vi "M3102A get data.vi"(5 "channel number":i32, 6 "TimeOut":i32, 7 "DAQpoints":i32, 8 "errorIn":errorcluster, 11 "moduleID":i32) -> (0 "errorOut":errorcluster, 2 "DAQdata":i16[](array[numeric]), 3 "moduleIDout":i32)   [LabVIEW 2021]
uses:
  <vilib>/Keysight_SD1/DAQ/base/DAQread_AIN.vi
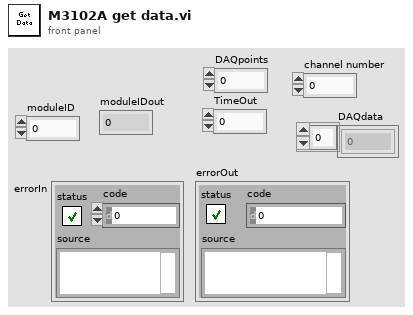
[diagram p1: front panel]
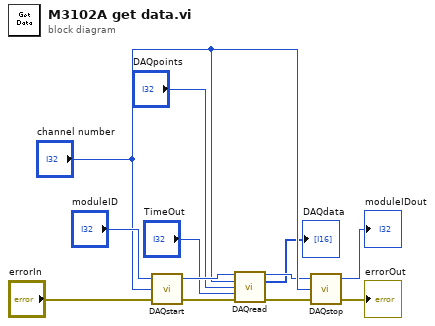
[diagram p0: block diagram]
diagram:
  n1 = call <vilib>:"DAQstart.vi"("errorIn"="errorIn", "nDAQ"="channel number", "moduleID"="moduleID") -> ("errorOut"=w12:errorcluster, "moduleIDout"=w11:i32)  [unwired: 1 in]
  n2 = call-poly <vilib>:"DAQread.vi"("moduleID"=w11, "nDAQ"="channel number", "DAQpoints"="DAQpoints", "TimeOut"="TimeOut", "errorIn"=w12) -> ("moduleIDout"=w3:i32, "DAQdata"=→"DAQdata":i16[], "errorOut"=w6:errorcluster)  [unwired: 8 in]
  n3 = call <vilib>:"DAQstop.vi"("errorIn"=w6, "nDAQ"="channel number", "moduleID"=w3) -> ("errorOut"=→"errorOut":errorcluster, "moduleIDout"=→"moduleIDout":i32)  [unwired: 1 in]
